vi "Motor Model.vi"(11 "Custom Motor Coefficients":T3={"Stall Torque"=0.71, "Stall Current"=134.0, "Free Speed"=18730.0, "Free Speed Current"=0.7, "Name"=""}) -> ()   [LabVIEW 2019]
doc: "Given the motor coefficients, compute the first order modeling factors."
uses:
  Motor Coefficients.ctl
  Motor Type.ctl
panel:
  out "Kv (rpm/V)":dbl format="%#_3p"
  in  "Motor Type":T1=enum."775 pro"
  out "Custom Motor Model Values":T2 {"Breaker" format="%#_3p"; "Kv" format="%#_3p"; "R" format="%#_3p"; "Kt" format="%#_3p"}
  out "Motor Curves":dbl[][](graph)
  # "Recommended use:\nClick the free-run button in toolbar. Choose the Motor Type."
  # "rpm"
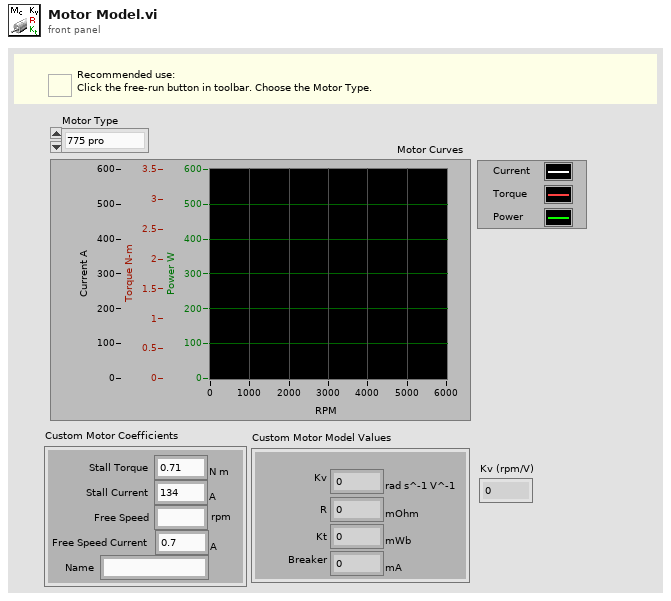
[diagram p1: front panel]
types:
  T1 = typedef "Motor Type.ctl" = enum16{"Custom", "775 pro", "CIM", "miniCIM", "Neo", "Neo 550", "Falcon 500"}
  T2 = cluster{"Kv":dbl[unit], "R":dbl[unit], "Kt":dbl[unit], "Breaker":dbl[unit]}
  T3 = typedef "Motor Coefficients.ctl" = cluster{"Stall Torque":dbl[unit], "Stall Current":dbl[unit], "Free Speed":dbl, "Free Speed Current":dbl[unit], "Name":string}
  T4 = typedef "Motor Operating Values.ctl" = cluster{"Kv":dbl[unit], "R":dbl[unit], "Kt":dbl[unit], "Breaker Size":dbl[unit]}
  T5 = typedef "LVRangeTypeDef.ctl" = cluster{"Minimum":dbl, "Maximum":dbl, "Increment":dbl, "Minor Increment":dbl, "Start":dbl}
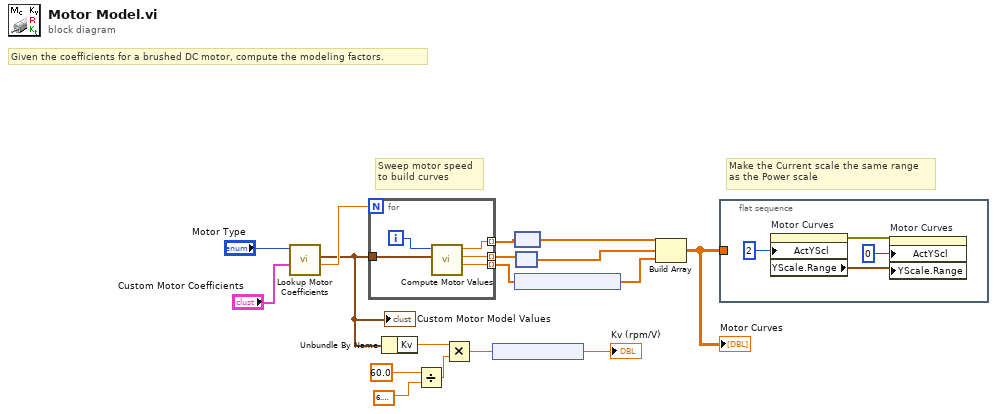
[diagram p0: block diagram]
diagram:
  # "Make the Current scale the same range\nas the Power scale"
  # "Sweep motor speed\nto build curves"
  # "Given the coefficients for a brushed DC motor, compute the modeling factors."
  n1 = call "Lookup Motor Coefficients.vi"("Custom Motor Coefficients"="Custom Motor Coefficients", "Motor Type"="Motor Type") -> ("Free Speed"=w16:dbl, "Motor Model Values"=w7:T4)  [unwired: 6 in, 2 out]
  "Custom Motor Model Values" <- w7
  n2 = for {
    N: w16 -> [_]
    tunnel: [w21] -> w15 mode=indexing
    tunnel: [w20] -> w13 mode=indexing
    tunnel: [w18] -> w12 mode=indexing
    tunnel: w7 -> [w19]
    i -> [w22]
    n3 = call "Compute Motor Values.vi"("Motor Model Values"=w19, "motor speed (rpm)"=w22) -> ("Power"=w18:dbl[unit], "Motor Torque"=w20:dbl[unit], "Current"=w21:dbl[unit])  [unwired: 6 in, 1 out]
  }
  n4 = Unbundle By Name(w7) -> ("Kv"=w6:dbl[unit])
  n5 = Divide(x=60.0, y=6.283185307179586) -> (x/y=w3:dbl)
  n6 = Multiply(x=w6, y=w3) -> (x*y=w2:dbl[unit])
  n7 = node(w2) -> (→"Kv (rpm/V)":dbl)
  n8 = node(w15) -> (w14:dbl[])
  n9 = node(w12) -> (w11:dbl[])
  n10 = node(w13) -> (w10:dbl[])
  n11 = Build Array(w14, w10, w11) -> (w8:dbl[][])
  "Motor Curves" <- w8
  n12 = flat-sequence {
    tunnel: w8 -> [_]
    frame #0 {
      n13 = property on="Motor Curves" class="WFGraph (strict)"("ActYScl"=2 ("Active Y Scale")) -> (error out=w24:errorcluster, "YScale.Range"=w23:T5)  [unwired: 2 in, 1 out]
      n14 = property on="Motor Curves" class="WFGraph (strict)"(error in=w24, "ActYScl"=0 ("Active Y Scale"), "YScale.Range"=w23) -> ()  [unwired: 1 in, 2 out]
    }
  }
